vi "Mcad15 regions.vi"(11 "file text in":string) -> (2 "Eval Regions":string[](array[string]), 3 "Regions":string[](array[string]))   [LabVIEW 2012, in "Design Server.lvlib"]
uses:
  Design Server.lvlib
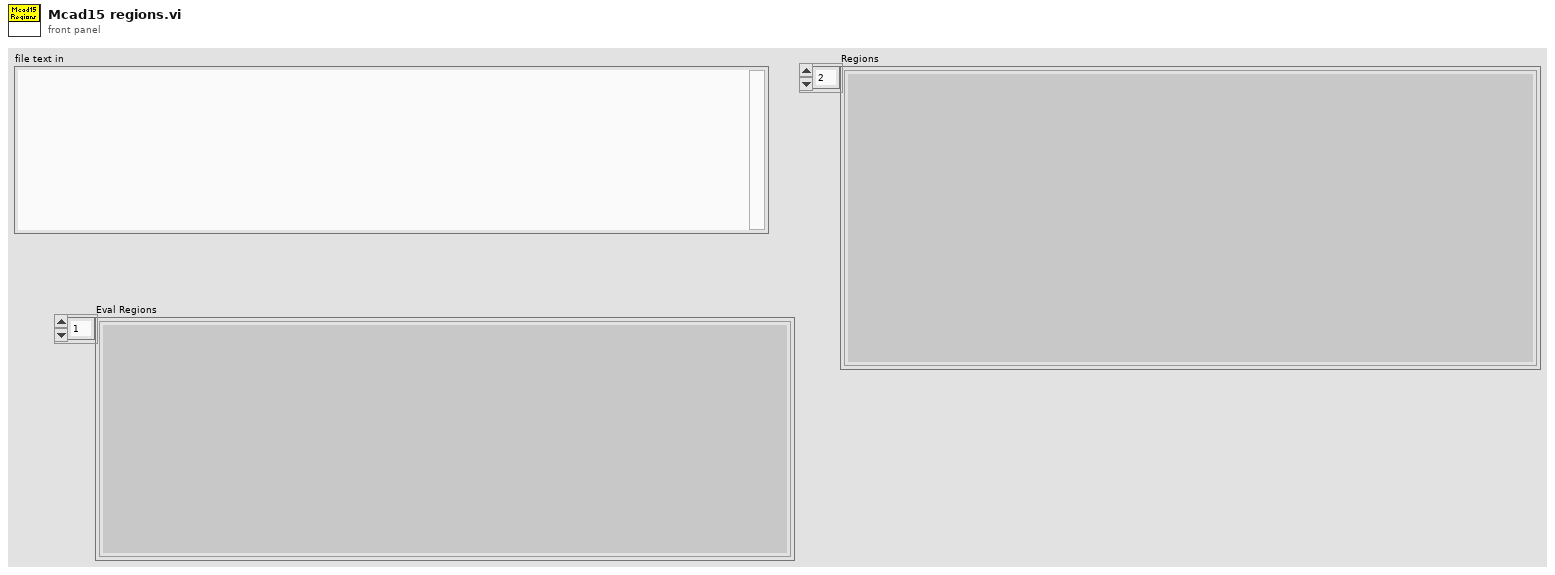
[diagram p1: front panel]
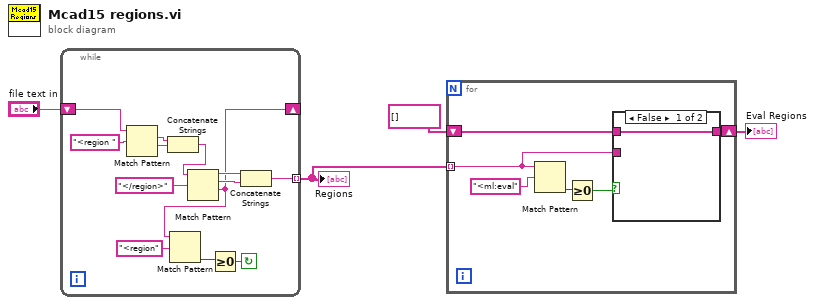
[diagram p0: block diagram]
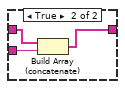
[diagram p2: hidden frame]
diagram:
  n1 = while {
    shift-right: [w8] -> _
    shift-left: "file text in" -> [w17]
    tunnel: [w9] -> w1 mode=indexing
    stop <- w6 continue-if-true
    n2 = Match Pattern(string=w17, regular expression="<region ") -> (match substring=w13:string, after substring=w12:string)  [unwired: 1 in, 2 out]
    n3 = Concatenate Strings(w13, w12) -> (w14:string)
    n4 = Match Pattern(string=w14, regular expression="</region>") -> (before substring=w11:string, match substring=w10:string, after substring=w8:string)  [unwired: 1 in, 1 out]
    n5 = Match Pattern(string=w8, regular expression="<region") -> (offset past match=w7:i32)  [unwired: 1 in, 3 out]
    n6 = Greater Or Equal To 0?(x=w7) -> (x >= 0?=w6:bool)
    n7 = Concatenate Strings(w11, w10) -> (w9:string)
  }
  "Regions" <- w1
  n8 = for {
    tunnel: w1 -> [w20] mode=indexing
    shift-right: [w19] -> w3
    shift-left: string[] [] -> [w18]
    n9 = Match Pattern(string=w20, regular expression="<ml:eval") -> (offset past match=w22:i32)  [unwired: 1 in, 3 out]
    n10 = Greater Or Equal To 0?(x=w22) -> (x >= 0?=w21:bool)
    n11 = case shown="False" w21 {
      tunnel: w20 -> [_ w27]
      tunnel: [w24 w26] -> w19
      tunnel: w18 -> [w24 w25]
      frame False {
      }
      frame True {
        n12 = Build Array (concatenate)(w25, w27) -> (w26:string[])
      }
    }
  }
  "Eval Regions" <- w3
